vi "Write iaa.vi"(8 "error in (no error)":errorcluster, 10 "iaa":dbl[unit] min=0.0 max=6.283185307179586, 11 "CurrentRotatorPositions in":refnum<class "CurrentRotatorPositions.lvclass">) -> (0 "error out":errorcluster, 3 "CurrentRotatorPositions out":refnum<class "CurrentRotatorPositions.lvclass">)   [LabVIEW 2014, in "TCSDataDefinitions.lvlib" / "TCSPublicStatus.lvlib" / "PointingPositions.lvlib" / "CurrentRotatorPositions.lvclass"]
uses:
  CurrentRotatorPositions.lvclass
  CurrentRotatorPositions.lvclass/CurrentRotatorPositions.ctl
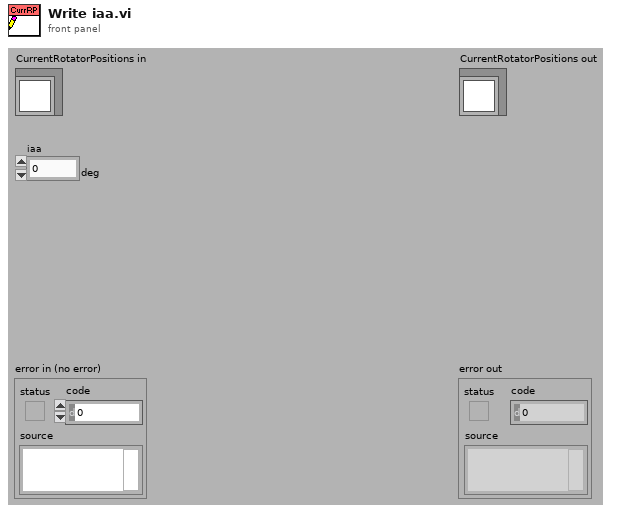
[diagram p1: front panel]
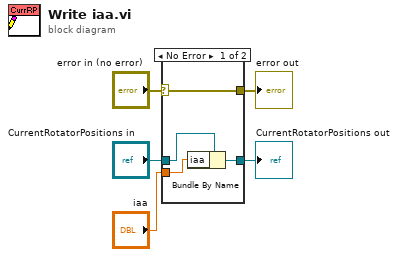
[diagram p0: block diagram]
diagram:
  n1 = case shown="No Error" "error in (no error)" {
    selector: "error in (no error)" -> [w9 w10]
    tunnel: [w9 w10] -> w4
    tunnel: [w7 w11] -> w2
    tunnel: "CurrentRotatorPositions in" -> [w8 w11]
    tunnel: "iaa" -> [w6 _]
    frame No Error {
      n2 = Bundle By Name(cluster=w8, "iaa"=w6) -> (w7:refnum<class "CurrentRotatorPositions.lvclass">)
    }
    frame Error {
    }
  }
  "error out" <- w4
  "CurrentRotatorPositions out" <- w2
